vi "Find Hysteresis Flow Index.vi"(2 "Value":string[][](array[string]), 3 "Current Step ID":i32) -> (1 "Hysteresis Step ID":i32)   [LabVIEW 2018]
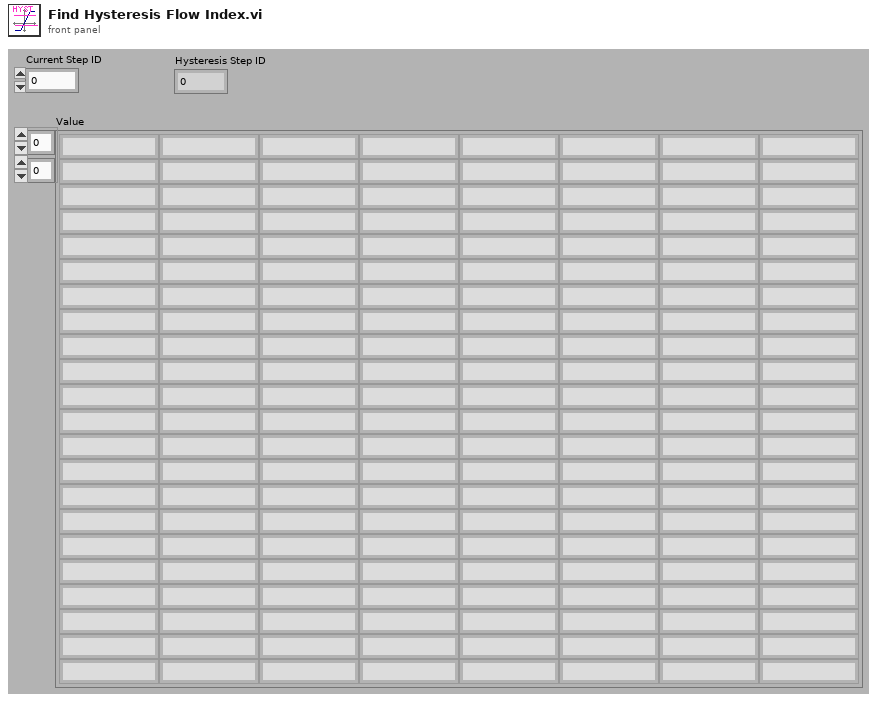
[diagram p1: front panel]
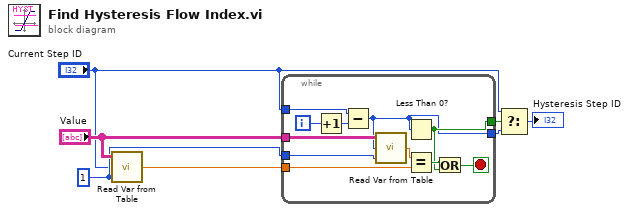
[diagram p0: block diagram]
diagram:
  w6 = 1 ("VAR Column Index")
  n1 = call "Read Var from Table.vi"("VAR Column Index"=w6, "Current Step ID"="Current Step ID", "Value"="Value") -> ("Numeric"=w5:dbl)
  n2 = while {
    tunnel: "Value" -> [w17]
    tunnel: "Current Step ID" -> [w16]
    tunnel: w6 -> [w15]
    tunnel: w5 -> [w12]
    tunnel: [w10] -> w4
    tunnel: [w9] -> w2
    i -> [w18]
    stop <- w11 stop-if-true
    n3 = Increment(x=w18) -> (x+1=w8:i32)
    n4 = Subtract(x=w16, y=w8) -> (x-y=w9:i32)
    n5 = call "Read Var from Table.vi"("VAR Column Index"=w15, "Current Step ID"=w9, "Value"=w17) -> ("Numeric"=w13:dbl)
    n6 = Less Than 0?(x=w9) -> (x < 0?=w10:bool)
    n7 = Equal?(x=w13, y=w12) -> (x = y?=w14:bool)
    n8 = Or(x=w14, y=w10) -> (x .or. y?=w11:bool)
  }
  n9 = Select(t="Current Step ID", s=w4, f=w2) -> (s? t:f=→"Hysteresis Step ID":i32)
